vi "Select Trace.vi"() -> ()   [LabVIEW 2014]
uses:
  <vilib>/Utility/file.llb/Read From Spreadsheet File (DBL).vi
  <vilib>/Utility/file.llb/Write To Spreadsheet File (DBL).vi
panel:
  in  "Select time pah":path
  out "All data (count)":dbl[][](array[numeric])
  in  "Tab Control":enum32{"Page 1", "Page 2", "Page 3"}(tab)
  out "XY Graph":cluster{dbl[], dbl[]}(graph)
  out "Waveform Graph":dbl[](graph)
  out "XY Graph 2":cluster{dbl[], dbl[]}(graph)
  out "time point":dbl[](array[numeric])
  out "Data rate":dbl
  in  "diff for binding one(nm)":dbl=0.654
  in  "Save?":bool
  out "Diff":dbl[](array[numeric])
  out "Array":dbl[](array[numeric])
  in  "Choose":i32
  out "All Selected Time (s)":dbl[][](array[numeric])
  out "All Selected Trace (nm)":dbl[][](array[numeric])
  in  "file path (dialog if empty)":path
  out "All end time":dbl[](array[numeric])
  out "All initial time":dbl[](array[numeric])
  out "Selected time intervals":dbl[][](array[numeric])=[[27.7, 33.5], [60.8, 67.5], [112.5, 115.5], [117.9, 123.6]]
  out "Time (s)":dbl[](array[numeric])
  out "xDNA (nm)":dbl[](array[numeric])
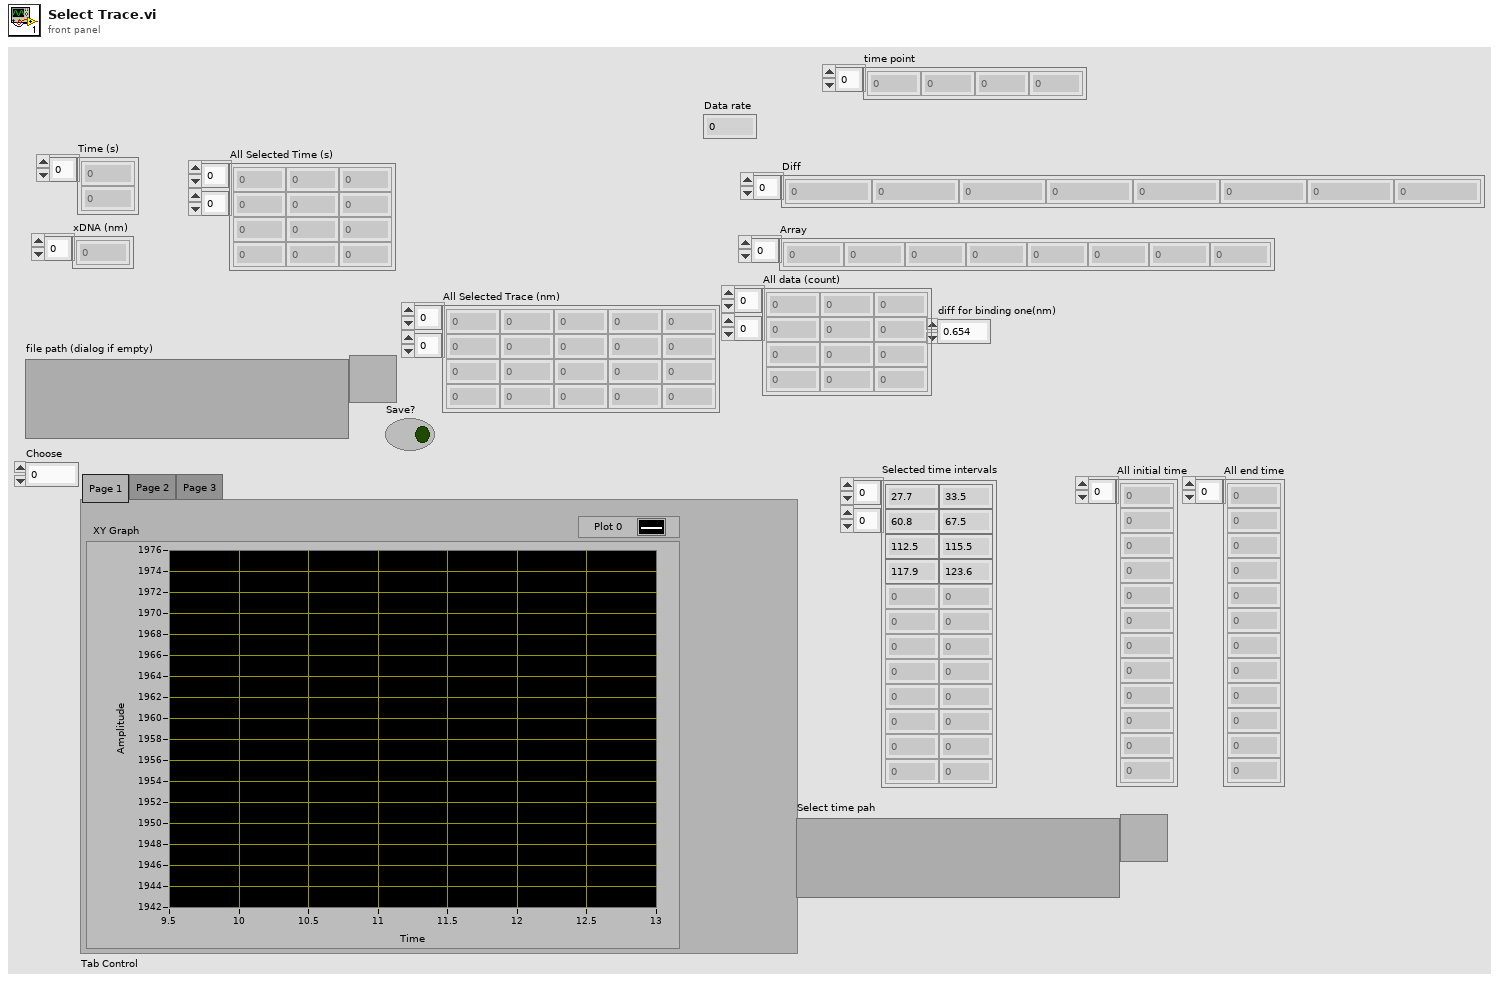
[diagram p1: front panel]
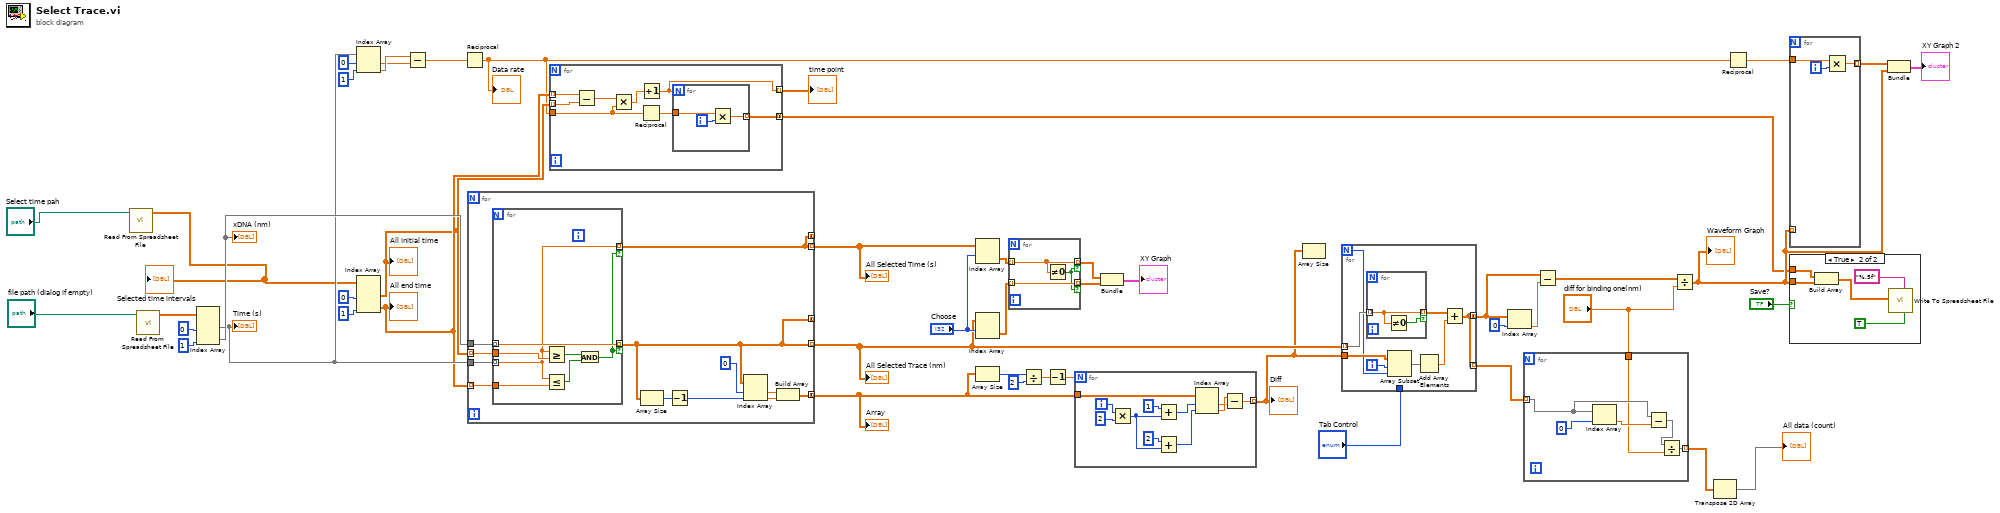
[diagram p0: block diagram]
diagram:
  n1 = call-poly <vilib>:"Read From Spreadsheet File.vi"("file path (dialog if empty)"="Select time pah") -> ("all rows"=w1:dbl[][])  [unwired: 6 in, 4 out]
  "Selected time intervals" <- w1
  n2 = call-poly <vilib>:"Read From Spreadsheet File.vi"("file path (dialog if empty)"="file path (dialog if empty)") -> ("all rows"=w45:dbl[][])  [unwired: 6 in, 4 out]
  n3 = Index Array(array=w45, index (col) #1=0 ("disabled index (col)"), index (col) #2=1 ("disabled index (col)")) -> (element #1=w22:dbl[], element #2=w42:dbl[])  [unwired: 2 in]
  "xDNA (nm)" <- w42
  "Time (s)" <- w22
  n4 = Index Array(array=w22, index #1=0 ("disabled index (col)"), index #2=1 ("disabled index (col)")) -> (element #1=w18:dbl, element #2=w19:dbl)
  n5 = Index Array(array=w1, index (col) #1=0 ("disabled index (col)"), index (col) #2=1 ("disabled index (col)")) -> (element #1=w11:dbl[], element #2=w12:dbl[])  [unwired: 2 in]
  "All initial time" <- w11
  "All end time" <- w12
  n6 = Subtract(x=w19, y=w18) -> (x-y=w13:dbl)
  n7 = Reciprocal(x=w13) -> (1/x=w10:dbl)
  "Data rate" <- w10
  n8 = for {
    tunnel: w22 -> [w60]
    tunnel: w42 -> [w59]
    tunnel: w11 -> [w58] mode=indexing
    tunnel: [w49] -> w29 mode=indexing
    tunnel: [w50] -> w41 mode=indexing
    tunnel: w12 -> [w57] mode=indexing
    tunnel: [w51] -> w34 mode=concatenating
    tunnel: [w50] -> _ mode=concatenating
    tunnel: [w49] -> _ mode=concatenating
    n9 = for {
      tunnel: w60 -> [w65] mode=indexing
      tunnel: w59 -> [w66] mode=indexing
      tunnel: w58 -> [w67]
      tunnel: [w66] -> w49 mode=indexing if=w61
      tunnel: [w65] -> w50 mode=indexing if=w61
      tunnel: w57 -> [w64]
      n10 = Greater Or Equal?(x=w65, y=w67) -> (x >= y?=w62:bool)
      n11 = Less Or Equal?(x=w65, y=w64) -> (x <= y?=w63:bool)
      n12 = And(x=w62, y=w63) -> (x .and. y?=w61:bool)
    }
    n13 = Array Size(array=w49) -> (size(s)=w55:i32)
    n14 = Decrement(x=w55) -> (x-1=w54:i32)
    n15 = Index Array(array=w49, index #1=0 ("index"), index #2=w54) -> (element #1=w53:dbl, element #2=w52:dbl)
    n16 = Build Array(w53, w52) -> (w51:dbl[])
  }
  "All Selected Trace (nm)" <- w29
  "All Selected Time (s)" <- w41
  "Array" <- w34
  n17 = for {
    tunnel: w12 -> [w75] mode=indexing
    tunnel: w11 -> [w74] mode=indexing
    tunnel: w10 -> [w70]
    tunnel: [w71] -> w9 mode=indexing
    tunnel: [w68] -> w8 mode=concatenating
    n18 = Subtract(x=w75, y=w74) -> (x-y=w73:dbl)
    n19 = Multiply(x=w73, y=w70) -> (x*y=w72:dbl)
    n20 = Reciprocal(x=w70) -> (1/x=w69:dbl)
    n21 = Increment(x=w72) -> (x+1=w71:dbl)
    n22 = for {
      N: w71 -> [_]
      tunnel: w69 -> [w77]
      tunnel: [w76] -> w68 mode=indexing
      i -> [w78]
      n23 = Multiply(x=w77, y=w78) -> (x*y=w76:dbl)
    }
  }
  "time point" <- w9
  n24 = Index Array(array=w41, index (row)="Choose") -> (element=w38:dbl[])  [unwired: 1 in]
  n25 = Index Array(array=w29, index (row)="Choose") -> (element=w36:dbl[])  [unwired: 1 in]
  n26 = Array Size(array=w34) -> (size(s)=w33:i32)
  n27 = for {
    tunnel: w38 -> [w80] mode=indexing
    tunnel: [w80] -> w37 mode=indexing if=w79
    tunnel: w36 -> [w81] mode=indexing
    tunnel: [w81] -> w35 mode=indexing if=w79
    n28 = Not Equal To 0?(x=w80) -> (x != 0?=w79:bool)
  }
  n29 = Divide(x=w33, y=2 ("index")) -> (x/y=w31:dbl)
  n30 = Decrement(x=w31) -> (x-1=w30:dbl)
  n31 = for {
    N: w30 -> [_]
    tunnel: w34 -> [w92]
    tunnel: [w89] -> w28 mode=indexing
    i -> [w87]
    n32 = Multiply(x=w87, y=2) -> (x*y=w85:i32)
    n33 = Add(x=1 ("y"), y=w85) -> (x+y=w86:i32)
    n34 = Add(x=2 ("y"), y=w85) -> (x+y=w84:i32)
    n35 = Index Array(array=w92, index #1=w86, index #2=w84) -> (element #1=w90:dbl, element #2=w91:dbl)
    n36 = Subtract(x=w91, y=w90) -> (x-y=w89:dbl)
  }
  "Diff" <- w28
  n37 = Bundle(w37, w35) -> (→"XY Graph":cluster{dbl[], dbl[]})  [unwired: 1 in]
  n38 = Array Size(array=w28) -> ()  [unwired: 1 out]
  n39 = for {
    N -> [w96]
    tunnel: w29 -> [w100] mode=indexing
    tunnel: w28 -> [w98]
    tunnel: [w93] -> w26 mode=concatenating
    tunnel: "Tab Control" -> [_]
    tunnel: [w93] -> w6 mode=indexing
    i -> [w97]
    n40 = for {
      tunnel: w100 -> [w101] mode=indexing
      tunnel: [w101] -> w99 mode=indexing if=w102
      n41 = Not Equal To 0?(x=w101) -> (x != 0?=w102:bool)
    }
    n42 = Array Subset(array=w98, index=w97, length=w96) -> (w95:dbl[])
    n43 = Add Array Elements(numeric array=w95) -> (sum=w94:dbl)
    n44 = Add(x=w99, y=w94) -> (x+y=w93:dbl[])
  }
  n45 = Index Array(array=w26, index=0) -> (element=w24:dbl)
  n46 = for {
    tunnel: w6 -> [w107] mode=indexing
    tunnel: "diff for binding one(nm)" -> [w105]
    tunnel: [w103] -> w4 mode=indexing
    n47 = Index Array(array=w107, index=0) -> (element=w106:dbl)
    n48 = Subtract(x=w107, y=w106) -> (x-y=w104:dbl[])
    n49 = Divide(x=w104, y=w105) -> (x/y=w103:dbl[])
  }
  n50 = Subtract(x=w26, y=w24) -> (x-y=w23:dbl[])
  n51 = Divide(x=w23, y="diff for binding one(nm)") -> (x/y=w15:dbl[])
  "Waveform Graph" <- w15
  n52 = Transpose 2D Array(2D array=w4) -> (transposed array=→"All data (count)":dbl[][])
  n53 = Reciprocal(x=w10) -> (1/x=w17:dbl)
  n54 = for {
    tunnel: w15 -> [_] mode=indexing
    tunnel: w17 -> [w110]
    tunnel: [w109] -> w16 mode=indexing
    i -> [w111]
    n55 = Multiply(x=w110, y=w111) -> (x*y=w109:dbl)
  }
  n56 = case shown="True" "Save?" {
    tunnel: w15 -> [_ w113]
    tunnel: w8 -> [_ w112]
    frame False {
    }
    frame True {
      n57 = Build Array(w112, w113) -> (w114:dbl[][])
      n58 = call-poly <vilib>:"Write To Spreadsheet File.vi"("transpose? (no:F)"=TRUE, "format (%.3f)"="%.5f", "2D data"=w114) -> ()  [unwired: 5 in, 1 out]
    }
  }
  n59 = Bundle(w16, w15) -> (→"XY Graph 2":cluster{dbl[], dbl[]})  [unwired: 1 in]
